vi "auto-ramp.vi"() -> ()   [LabVIEW 2012, in "Mecanum Drive.lvrbt"]
uses:
  Mecanum Drive.lvrbt
  <vilib>/NXT/HiTechnic/HiTechnic Controls/HiTechnic Port.ctl
  <vilib>/NXT/Block Support/NXT_InputPort.ctl
  SubVIs/auto_drive_TYP.ctl
  <vilib>/NXT/Hardware/Plugins/Tetrix DC Motor/TetrixDCMotorAddress.ctl
  <vilib>/NXT/Dual Mode Library/Waits/Wait_Num(msec).vi
  <vilib>/NXT/NXTIO Xnodes/NXTIONodeSubVIs/TETRIX IO Check Battery.vi
  <vilib>/NXT/NXTIO Xnodes/NXTIONodeSubVIs/TETRIX IO Stop DC Motors.vi
  <vilib>/NXT/Subs/LVHSConnector.ctl
  <vilib>/NXT/NXTIO Xnodes/AddressXNode/NXTIOAddress.xnode
  <vilib>/NXT/NXTIO Xnodes/NXTIOXNode/NXTIO.xnode
  <vilib>/NXT/LegoClasses/BrickReference/BrickReference.lvclass
panel:
  out "Enabled":bool
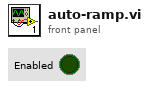
[diagram p1: front panel]
types:
  T1 = typedef "auto_drive_TYP.ctl" = cluster{"Left X":i8, "Left Y":i8, "Right X":i8, "Power (100)":i8, "Wait (ms)":u32, "Enc/Deg Target":i32, "Move Type":enum16{"Relative Degrees", "Wait", "Encoder"}}
  T2 = typedef "HiTechnic Port.ctl" = cluster{"Port":T3, "MUX Port":u8}
  T3 = typedef "NXT_InputPort.ctl" = u32
  T4 = typedef "TetrixDCMotorAddress.ctl" = i32
  T5 = typedef "LVHSConnector.ctl" = refnum<class "BrickReference.lvclass">
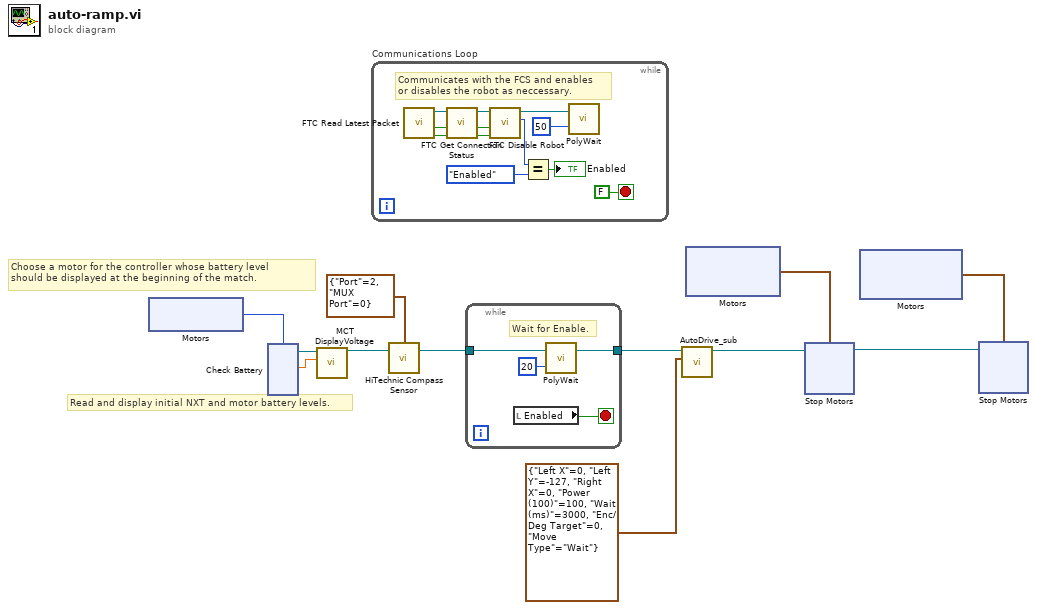
[diagram p0: block diagram]
diagram:
  # "Read and display initial NXT and motor battery levels."
  # "Choose a motor for the controller whose battery level \nshould be displayed at the beginning of the match."
  n1 = xnode "Motors"() -> ("Motor"=w10:T4)
  n2 = xnode "Check Battery"("Motors"=w10) -> ("Voltage 1"=w11:sgl, "NXT/EV3"=w12:T5)  [unwired: 1 in]
  n3 = call <vilib>:"MCT DisplayVoltage.vi"("Motor Voltage"=w11, "NXT"=w12) -> ("NXT"=w8:T5)  [unwired: 9 in]
  n4 = while "Communications Loop" {
    stop <- FALSE stop-if-true
    # "Communicates with the FCS and enables \nor disables the robot as neccessary."
    n5 = call <vilib>:"FTC Read Latest Packet.vi"() -> ("Packet Received?"=w22:bool, "Stopped?"=w21:bool, "NXT"=w24:T5)  [unwired: 6 in, 3 out]
    n6 = call <vilib>:"FTC Get Connection Status.vi"("Packet Received?"=w22, "Stopped?"=w21, "NXT"=w24) -> ("Online?"=w13:bool, "Stopped?"=w14:bool, "NXT"=w23:T5)  [unwired: 5 in]
    n7 = call <vilib>:"FTC Disable Robot.vi"("Online?"=w13, "Stopped?"=w14, "NXT"=w23) -> ("Enabled?"=w17:enum16{"Disabled", "Enabled"}, "NXT"=w19:T5)  [unwired: 3 in]
    n8 = Equal?(x=w17, y=enum16{"Disabled", "Enabled"}."Enabled") -> (x = y?=→"Enabled":bool)
    n9 = call-poly <vilib>:"PolyWait.vi"("Time (100 msec)"=u32 50 ("Time (msec)"), "NXT/EV3"=w19) -> ()  [unwired: 2 in, 1 out]
  }
  n10 = call <vilib>:"HiTechnic Compass Sensor.vi"("NXT/EV3"=w8, "Port/MUX"=T2 {"Port"=2, "MUX Port"=0}) -> ("NXT/EV3"=w7:T5)  [unwired: 1 in, 1 out]
  n11 = while {
    tunnel: [w26] -> w6
    tunnel: w7 -> [w25]
    stop <- w27 stop-if-true
    # "Wait for Enable."
    n12 = local read "Enabled"() -> (w27:bool)
    n13 = call-poly <vilib>:"PolyWait.vi"("Time (100 msec)"=u32 20 ("Time (msec)"), "NXT/EV3"=w25) -> ("NXT/EV3"=w26:T5)  [unwired: 2 in]
  }
  n14 = call "AutoDrive_sub.vi"("Drive Control"=T1 {"Left X"=0, "Left Y"=-127, "Right X"=0, "Power (100)"=100, "Wait (ms)"=3000, "Enc/Deg Target"=0, "Move Type"=enum."Wait"}, "NXT/EV3"=w6) -> ("NXT/EV3 out"=w3:T5)  [unwired: 8 in, 1 out]
  n15 = xnode "Motors"() -> ("Motor"=w4:cluster{"TetrixDCMotor":T4, "TetrixDCMotor":T4})
  n16 = xnode "Stop Motors"("Motors"=w4, "NXT/EV3"=w3) -> ("NXT/EV3"=w1:T5)
  n17 = xnode "Motors"() -> ("Motor"=w2:cluster{"TetrixDCMotor":T4, "TetrixDCMotor":T4})
  n18 = xnode "Stop Motors"("Motors"=w2, "NXT/EV3"=w1) -> ()  [unwired: 1 out]
